vi "findSpectrometer.vi"(8 "error in (no error)":errorcluster, 11 "SEDSpectrometer in":refnum<class "SEDSpectrometer.lvclass">) -> (0 "error out":errorcluster, 1 "NumOfDevices":i32, 2 "AviableSpec":u8[](array[numeric]), 3 "SEDSpectrometer out":refnum<class "SEDSpectrometer.lvclass">)   [LabVIEW 2016, in "SEDSpectrometer.lvclass"]
uses:
  SEDSpectrometer.lvclass
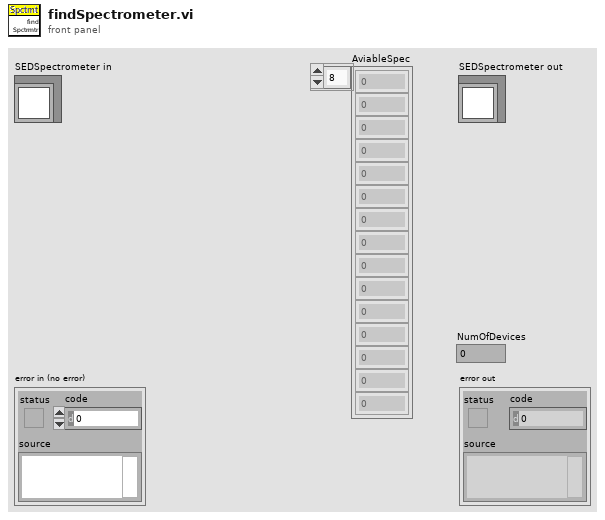
[diagram p1: front panel]
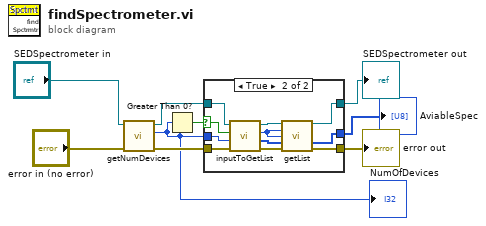
[diagram p0: block diagram]
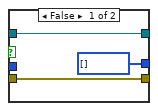
[diagram p2: hidden frame]
diagram:
  n1 = call "getNumDevices.vi"("error in (no error)"="error in (no error)", "SEDSpectrometer in"="SEDSpectrometer in") -> ("error out"=w5:errorcluster, "Output Value"=w1:i32, "SEDSpectrometer out"=w6:refnum<class "SEDSpectrometer.lvclass">)  [unwired: 7 in]
  "NumOfDevices" <- w1
  n2 = Greater Than 0?(x=w1) -> (x > 0?=w7:bool)
  n3 = case shown="True" w7 {
    selector: w7 -> [_ w21]
    tunnel: w6 -> [w11 w23]
    tunnel: w1 -> [_ w20]
    tunnel: w5 -> [w10 w19]
    tunnel: [u8[] [] w15] -> w2
    tunnel: [w11 w14] -> w4
    tunnel: [w10 w13] -> w3
    frame False {
    }
    frame True {
      n4 = call "inputToGetList.vi"("error in (no error)"=w19, "NumOfDevices"=w20, "DeviceConnected"=w21, "SEDSpectrometer in"=w23) -> ("error out"=w18:errorcluster, "ListInput"=w16:u8[], "ListSizeInput"=w17:i32, "SEDSpectrometer out"=w22:refnum<class "SEDSpectrometer.lvclass">)  [unwired: 4 in]
      n5 = call "getList.vi"("SEDSpectrometer in"=w22, "ListSizeInput"=w17, "RequiredSizeInput"=w17, "ListInpit"=w16, "error in (no error)"=w18) -> ("SEDSpectrometer out"=w14:refnum<class "SEDSpectrometer.lvclass">, "List Output"=w15:u8[], "error out"=w13:errorcluster)  [unwired: 8 in]
    }
  }
  "error out" <- w3
  "SEDSpectrometer out" <- w4
  "AviableSpec" <- w2
